vi "1820 Sweep ETA.vi"(8 "Power Supply Field (T)":dbl, 9 "Target Field Rate (T/min)":dbl, 10 "Magnet Field (T)":dbl, 11 "Target Field (T)":dbl) -> (1 "Remaining Time (sec)":dbl, 2 "ETA string":string, 3 "ETA timestamp":timestamp)   [LabVIEW 2019, in "Instrument.Oxford1820.lvclass"]
uses:
  Instrument.Oxford1820.lvclass
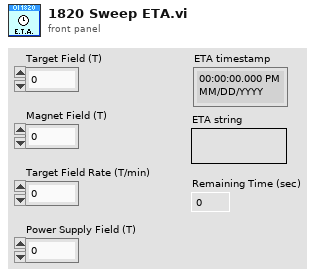
[diagram p1: front panel]
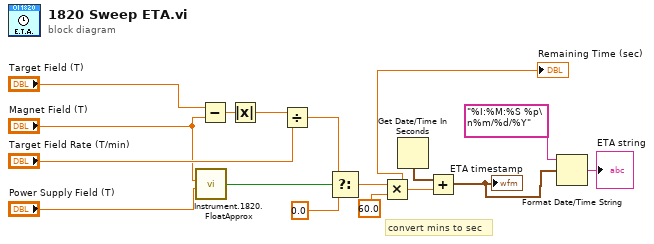
[diagram p0: block diagram]
diagram:
  # "convert mins to sec"
  n1 = call "Instrument.1820.FloatApprox.vi"("y"="Power Supply Field (T)", "x"="Magnet Field (T)") -> ("x ~ y?"=w10:bool)  [unwired: 4 in]
  n2 = Subtract(x="Target Field (T)", y="Magnet Field (T)") -> (x-y=w12:dbl)
  n3 = Absolute Value(x=w12) -> (abs(x)=w5:dbl)
  n4 = Divide(x=w5, y="Target Field Rate (T/min)") -> (x/y=w15:dbl)
  n5 = Select(t=w15, s=w10, f=0.0) -> (s? t:f=w7:dbl)
  n6 = Multiply(x=w7, y=60.0 ("f")) -> (x*y=w4:dbl)
  "Remaining Time (sec)" <- w4
  n7 = Get Date/Time In Seconds() -> (seconds since 1Jan1904=w9:timestamp)
  n8 = Add(x=w9, y=w4) -> (x+y=w1:timestamp)
  "ETA timestamp" <- w1
  n9 = Format Date/Time String(time format string (%c)="%I:%M:%S %p\n%m/%d/%Y", seconds (now)=w1) -> (date/time string=→"ETA string":string)  [unwired: 1 in]
